vi "ExSubSetSpeFileHeader.vi"(5 "error in (no error)":errorcluster, 6 "Pulser Handle":u32, 7 "Calibration Handle":u32, 8 "Camera Handle":u32, 9 "File Handle":u32) -> (0 "Pulser Handle":u32, 1 "Calibration Handle":u32, 2 "Camera Handle":u32, 3 "File Handle":u32, 4 "error out":errorcluster)   [LabVIEW 2010]
panel:
  # "ExSubSetSpeFileHeader.vi\nThis VI will use information from other device handles to set \ninformation in a file header.  Note that this is only valid for\nSPE file types at this time.  Device handles other than the File Handle are\noptional and the user may enter any information manually if desired.\nHeader information is NOT saved to the file until a Data Write (FileSaveData.vi)\nis done or the file is Closed (FileClose.vi)."
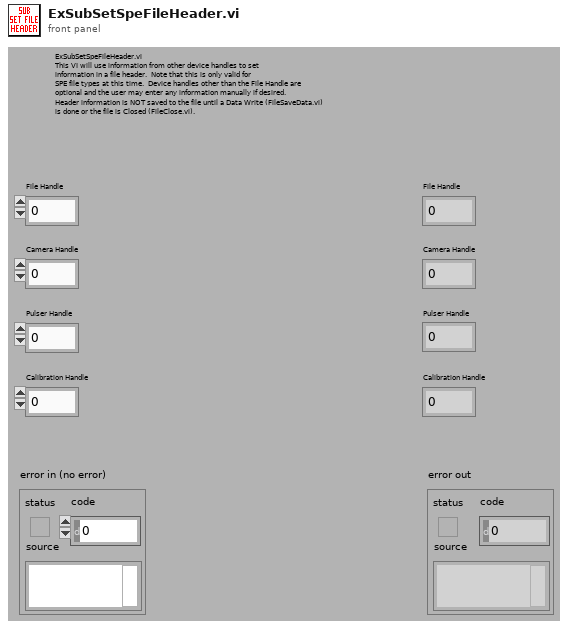
[diagram p1: front panel]
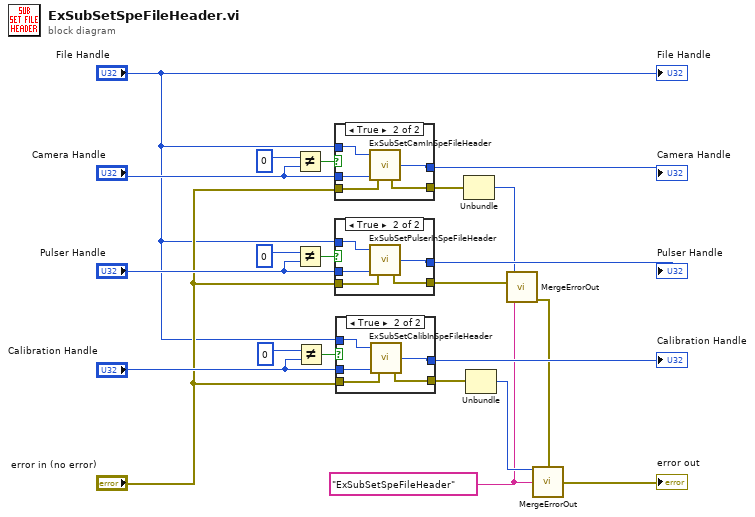
[diagram p0: block diagram]
diagram:
  w2 = "ExSubSetSpeFileHeader"
  n1 = Not Equal?(x=0, y="Camera Handle") -> (x != y?=w22:bool)
  n2 = Not Equal?(x=0, y="Pulser Handle") -> (x != y?=w18:bool)
  n3 = Not Equal?(x=0, y="Calibration Handle") -> (x != y?=w11:bool)
  n4 = case shown="True" w22 {
    tunnel: "File Handle" -> [_ w29]
    tunnel: "Camera Handle" -> [w24 w28]
    tunnel: [w24 w26] -> w19
    tunnel: "error in (no error)" -> [w23 w27]
    tunnel: [w23 w25] -> w14
    frame False {
    }
    frame True {
      n5 = call "ExSubSetCamInSpeFileHeader.vi"("error in (no error)"=w27, "Camera Handle"=w28, "File Handle"=w29) -> ("error out"=w25:errorcluster, "Camera Handle"=w26:u32)  [unwired: 1 out]
    }
  }
  "Camera Handle" <- w19
  n6 = case shown="True" w18 {
    tunnel: "File Handle" -> [_ w36]
    tunnel: "Pulser Handle" -> [w31 w35]
    tunnel: [w31 w33] -> w15
    tunnel: "error in (no error)" -> [w30 w34]
    tunnel: [w30 w32] -> w12
    frame False {
    }
    frame True {
      n7 = call "ExSubSetPulserInSpeFileHeader.vi"("error in (no error)"=w34, "Pulser Handle"=w35, "File Handle"=w36) -> ("error out"=w32:errorcluster, "Pulser Handle"=w33:u32)  [unwired: 1 out]
    }
  }
  "Pulser Handle" <- w15
  n8 = case shown="True" w11 {
    tunnel: "File Handle" -> [_ w43]
    tunnel: "Calibration Handle" -> [w38 w42]
    tunnel: [w38 w40] -> w7
    tunnel: "error in (no error)" -> [w37 w41]
    tunnel: [w37 w39] -> w6
    frame False {
    }
    frame True {
      n9 = call "ExSubSetCalibInSpeFileHeader.vi"("error in (no error)"=w41, "Calibration Handle"=w42, "File Handle"=w43) -> ("error out"=w39:errorcluster, "Calibration Handle"=w40:u32)  [unwired: 1 out]
    }
  }
  "Calibration Handle" <- w7
  n10 = Unbundle(w14) -> ("code"=w13:i32)  [unwired: 2 out]
  n11 = Unbundle(w6) -> ("code"=w5:i32)  [unwired: 2 out]
  n12 = call <userlib>:"MergeErrorOut.vi"("error in"=w12, "Fucntion Name"=w2, "ErrorCode"=w13) -> ("error out"=w4:errorcluster)
  n13 = call <userlib>:"MergeErrorOut.vi"("error in"=w4, "Fucntion Name"=w2, "ErrorCode"=w5) -> ("error out"=→"error out":errorcluster)
  "File Handle" <- "File Handle"
